vi "Constant Output Averager.vi"(0 "Init(T)/Run(F)":bool, 5 "AveWidth":i32, 7 "Input":fxp<+/-,32,16>) -> (8 "Output":fxp<+/-,62,46>, 15 "VerMult":fxp<+,20,20>)   [LabVIEW 2013]
uses:
  <vilib>/rvi/FXPMathLib/FxpDiv/subVIs/nifxpmath_Div_SimConfig.ctl
  <vilib>/rvi/Emulation/niFpgaSctlEmulationGetInTimedLoop.vi
  <vilib>/rvi/Emulation/niFpgaEmulationReportErrorSimple.vi
  <vilib>/rvi/Emulation/niFpgaGetClockAttributes.vi
  <vilib>/rvi/FXPMathLib/FxpDiv/simVIs/DllFxpDivTemp_sub.vi
  <vilib>/rvi/Emulation/niFpgaCriticalErrorInLSC.vi
  <vilib>/rvi/FXPMathLib/FxpDiv/XNode/nifxpmath_Div.xnode
  <vilib>/rvi/FXPMathLib/FxpSub/XNode/nifxpmath_Sub.xnode
  <vilib>/rvi/FXPMathLib/FxpAdd/XNode/nifxpmath_Add.xnode
  <vilib>/rvi/FXPMathLib/FxpMul/XNode/nifxpmath_Multiplier.xnode
  <vilib>/rvi/FXPMathLib/sim/FxpSim.dll
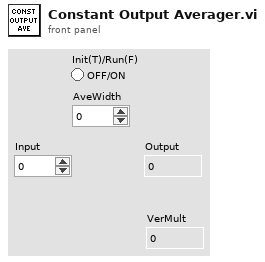
[diagram p1: front panel]
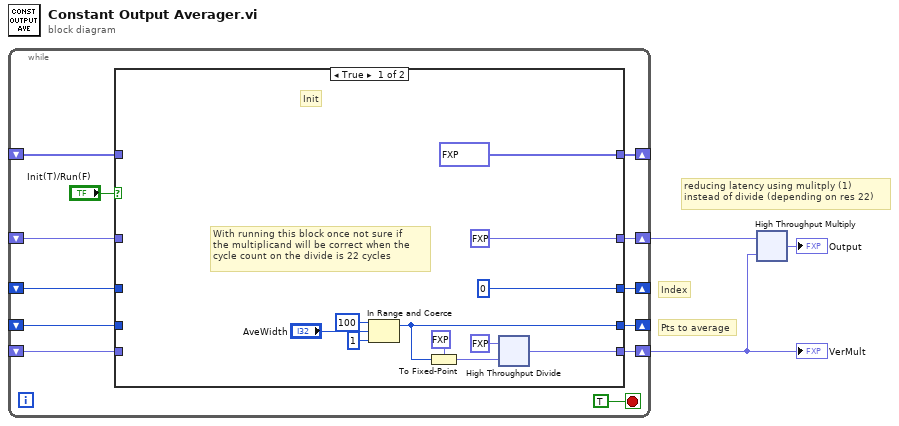
[diagram p0: block diagram]
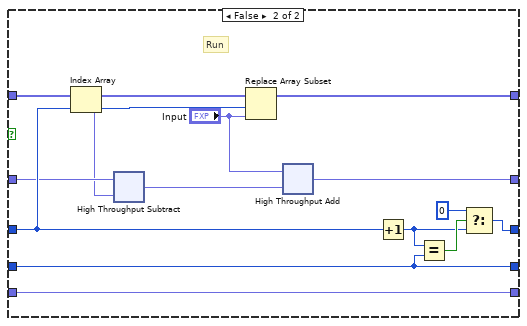
[diagram p2: hidden frame]
diagram:
  # "reducing latency using mulitply (1)\ninstead of divide (depending on res 22)"
  # "Pts to average"
  # "Index"
  n1 = while {
    shift-right: [w14] -> _
    shift-left: _ -> [w13]
    shift-right: [w10] -> _
    shift-left: _ -> [w8]
    shift-right: [w12] -> w3
    shift-left: _ -> [w6]
    shift-right: [w9] -> _
    shift-left: _ -> [w7]
    shift-right: [w5] -> w2
    shift-left: _ -> [w4]
    stop <- TRUE stop-if-true
    n2 = case shown="True" "Init(T)/Run(F)" {
      tunnel: [fxp<+/-,32,16>[] [0.0, 0.0, 0.0, 0.0, 0.0, 0.0, 0.0, 0.0, 0.0, 0.0, 0.0, 0.0, 0.0, 0.0, 0.0, 0.0, 0.0, 0.0, 0.0, 0.0, 0.0, 0.0, 0.0, 0.0, 0.0, 0.0, 0.0, 0.0, 0.0, 0.0, 0.0, 0.0, 0.0, 0.0, 0.0, 0.0, 0.0, 0.0, 0.0, 0.0, 0.0, 0.0, 0.0, 0.0, 0.0, 0.0, 0.0, 0.0, 0.0, 0.0, 0.0, 0.0, 0.0, 0.0, 0.0, 0.0, 0.0, 0.0, 0.0, 0.0, 0.0, 0.0, 0.0, 0.0, 0.0, 0.0, 0.0, 0.0, 0.0, 0.0, 0.0, 0.0, 0.0, 0.0, 0.0, 0.0, 0.0, 0.0, 0.0, 0.0, 0.0, 0.0, 0.0, 0.0, 0.0, 0.0, 0.0, 0.0, 0.0, 0.0, 0.0, 0.0, 0.0, 0.0, 0.0, 0.0, 0.0, 0.0, 0.0, 0.0] w56] -> w14
      tunnel: w13 -> [_ w67]
      tunnel: [fxp<+/-,42,26> 0.0 w55] -> w12
      tunnel: [0 w61] -> w10
      tunnel: [w19 w65] -> w9
      tunnel: w8 -> [_ w66]
      tunnel: w7 -> [_ w65]
      tunnel: w6 -> [_ w60]
      tunnel: [w16 w54] -> w5
      tunnel: w4 -> [_ w54]
      frame True {
        # "With running this block once not sure if\nthe multiplicand will be correct when the\ncycle count on the divide is 22 cycles"
        # "Init"
        n3 = In Range and Coerce(upper limit=100, x="AveWidth", lower limit=1) -> (coerced(x)=w19:i32)  [unwired: 1 out]
        n4 = To Fixed-Point(fixed-point type=fxp<+,7,7> 0.0 ("fixed-point"), number=w19) -> (fixed-point=w18:fxp<+,7,7>)
        n5 = xnode "High Throughput Divide"("x"=fxp<+,1,1> 1.0, "y"=w18) -> ("x/y"=w16:fxp<+,20,20>)
      }
      frame False {
        # "Run"
        n6 = Index Array(array=w67, index=w66) -> (element=w59:fxp<+/-,32,16>)
        n7 = xnode "High Throughput Subtract"("x"=w60, "y"=w59) -> ("x-y"=w58:fxp<+/-,42,26>)
        n8 = Replace Array Subset(array=w67, new element="Input", index=w66) -> (w56:fxp<+/-,32,16>[])
        n9 = xnode ("High Throughput Add")("x"="Input", "y"=w58) -> ("x+y"=w55:fxp<+/-,42,26>)
        n10 = Increment(x=w66) -> (x+1=w63:i32)
        n11 = Equal?(x=w63, y=w65) -> (x = y?=w64:bool)
        n12 = Select(t=0, s=w64, f=w63) -> (s? t:f=w61:i32)
      }
    }
  }
  "VerMult" <- w2
  n13 = xnode "High Throughput Multiply"("x"=w3, "y"=w2) -> ("x*y"=→"Output":fxp<+/-,62,46>)
